vi "Resize Tree Columns.vi"(8 "error in":errorcluster, 10 "Number of columns":i32, 11 "TreeControl ref in":refnum<vi>) -> (0 "error out":errorcluster)   [LabVIEW 2019]
doc: "This VI resizes the last column in a tree, so that only specified number of columns are visible"
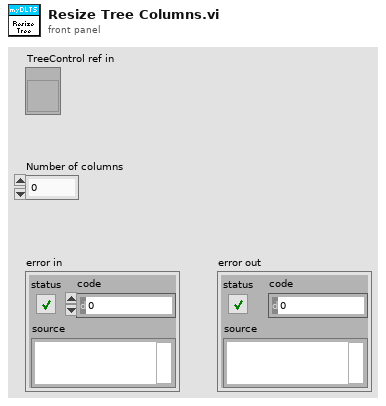
[diagram p1: front panel]
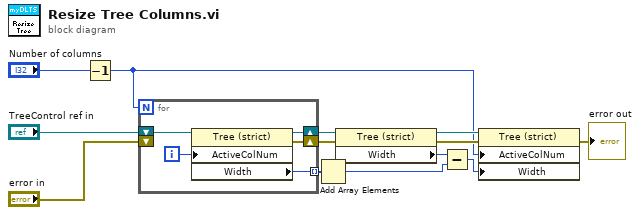
[diagram p0: block diagram]
diagram:
  n1 = Decrement(x="Number of columns") -> (x-1=w2:i32)
  n2 = for {
    N: w2 -> [_]
    shift-right: [w16] -> w8
    shift-left: "TreeControl ref in" -> [w18]
    tunnel: [w15] -> w9 mode=indexing
    shift-right: [w14] -> w7
    shift-left: "error in" -> [_]
    i -> [w17]
    n3 = property on="Property Node" class="Tree (strict)"(reference=w18, "ActiveColNum"=w17) -> (reference out=w16:refnum<vi>, error out=w14:errorcluster, "Width"=w15:i32)  [unwired: 1 in]
  }
  n4 = Add Array Elements(numeric array=w9) -> (sum=w11:i32)
  n5 = property on="Property Node" class="Tree (strict)"(reference=w8, error in=w7) -> (reference out=w13:refnum<vi>, error out=w6:errorcluster, "Width"=w10:u32)
  n6 = Subtract(x=w10, y=w11) -> (x-y=w12:u32)
  n7 = property on="Property Node" class="Tree (strict)"(reference=w13, error in=w6, "ActiveColNum"=w2, "Width"=w12) -> (error out=→"error out":errorcluster)  [unwired: 1 out]
